vi "Page_Source_Can_Add_To_Bottom.vi"(8 "error in (no error)":errorcluster, 11 "AB_Source in":refnum<class "AB_Source.lvclass">) -> (0 "error out":errorcluster, 1 "message":string, 2 "canAddToBottom":bool, 3 "AB_Source out":refnum<class "AB_Source.lvclass">)   [LabVIEW 2020, in "AB_Source.lvclass"]
uses:
  <vilib>/AppBuilder/AB_Classes/Source/AB_Source.lvclass
  <vilib>/AppBuilder/AB_Classes/Source/AB_Source.lvclass/AB_Source.ctl
  <resource>/Framework/Providers/Common/provcom_StringGlobals.vi
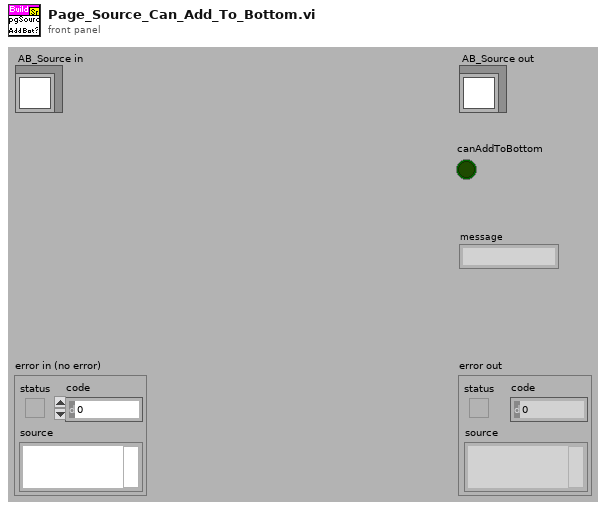
[diagram p1: front panel]
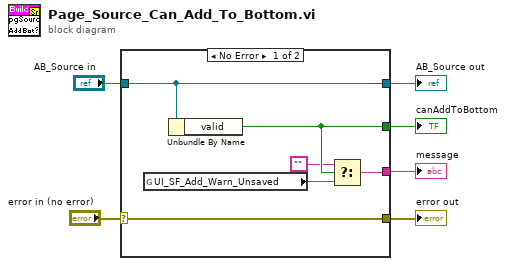
[diagram p0: block diagram]
diagram:
  n1 = case shown="No Error" "error in (no error)" {
    selector: "error in (no error)" -> [w12 w14]
    tunnel: [w12 w14] -> w5
    tunnel: [w11 w13] -> w3
    tunnel: "AB_Source in" -> [w11 w13]
    tunnel: [w10 _] -> w2
    tunnel: [w7 _] -> w1
    frame No Error {
      n2 = global read "provcom_StringGlobals.vi" "UI_SF_Add_Warn_Unsaved"() -> (w8:string)
      n3 = Unbundle By Name(w11) -> ("valid"=w10:bool)
      n4 = Select(t="", s=w10, f=w8) -> (s? t:f=w7:string)
    }
    frame Error {
    }
  }
  "error out" <- w5
  "AB_Source out" <- w3
  "canAddToBottom" <- w2
  "message" <- w1
